vi "Find the extremal value using 2nd polynomial given X and Y.vi"(5 "initial guess index of X":dbl, 6 "Y":dbl[](array[numeric]), 7 "X":dbl[](array[numeric])) -> (0 "Best Fit":cluster{"X":dbl[], "Best Polynomial Fit":dbl[]}, 1 "Xm":dbl, 3 "input":cluster{"X":dbl[], "Best Polynomial Fit":dbl[]})   [LabVIEW 2014]
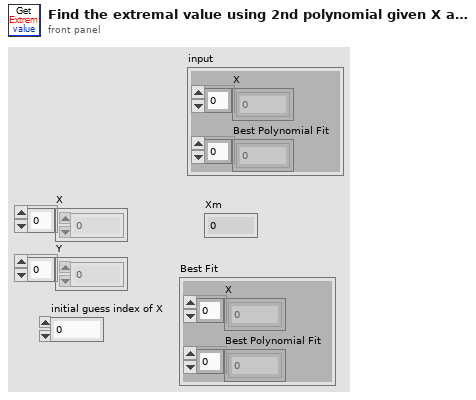
[diagram p1: front panel]
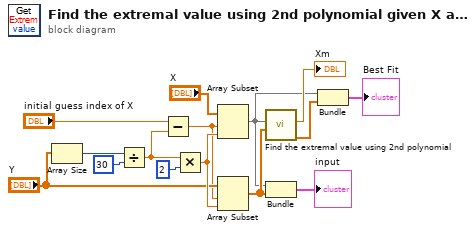
[diagram p0: block diagram]
diagram:
  n1 = Array Size(array="Y") -> (size(s)=w10:i32)
  n2 = Divide(x=w10, y=30) -> (x/y=w5:dbl)
  n3 = Subtract(x="initial guess index of X", y=w5) -> (x-y=w4:dbl)
  n4 = Multiply(x=w5, y=2) -> (x*y=w14:dbl)
  n5 = Array Subset(array="X", index=w4, length=w14) -> (w1:dbl[])
  n6 = Array Subset(array="Y", index=w4, length=w14) -> (w2:dbl[])
  n7 = call "Find the extremal value using 2nd polynomial.vi"("Y"=w2, "X"=w1) -> ("Best Polynomial Fit"=w8:dbl[], "Xm"=→"Xm":dbl)  [unwired: 3 in, 1 out]
  n8 = Bundle(w1, w2) -> (→"input":cluster{dbl[], dbl[]})  [unwired: 1 in]
  n9 = Bundle(w1, "Best Polynomial Fit"=w8) -> (→"Best Fit":cluster{dbl[], "Best Polynomial Fit":dbl[]})  [unwired: 1 in]
